vi "road to next map.vi"(7 "Numeric in":i32) -> (8 "Numeric out":i32)   [LabVIEW 2010]
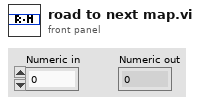
[diagram p1: front panel]
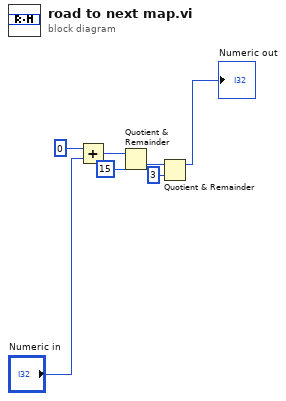
[diagram p0: block diagram]
diagram:
  n1 = Add(x=0, y="Numeric in") -> (x+y=w3:i32)
  n2 = Quotient & Remainder(x=w3, y=15) -> (floor(x/y)=w5:i32)  [unwired: 1 out]
  n3 = Quotient & Remainder(x=w5, y=3) -> (x-y*floor(x/y)=→"Numeric out":i32)  [unwired: 1 out]
